vi "TOP-调试与报错.vi"(7 "枚举-错误类型":T1, 8 "错误 i":errorcluster, 11 "输入":variant) -> (0 "错误 o":errorcluster, 3 "输出":variant)   [LabVIEW 2017, in "调试与报错.lvlib"]
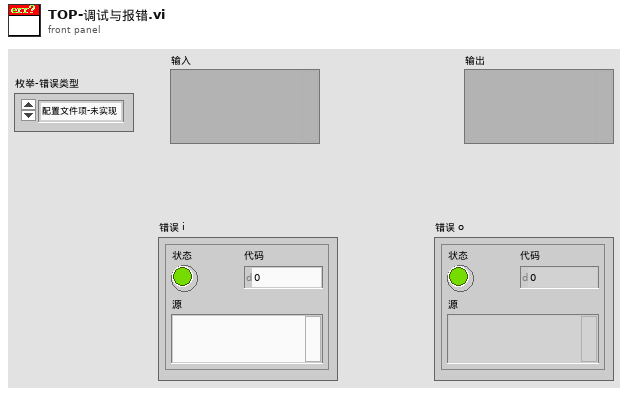
[diagram p1: front panel]
types:
  T1 = typedef "调试与报错.lvlib/枚举-错误类型.ctl" = enum16{"配置文件项-未实现", "路径-未实现"}
  T2 = typedef "调试与报错.lvlib/簇-输入-配置文件项未实现.ctl" = cluster{"段名":string, "键名":string}
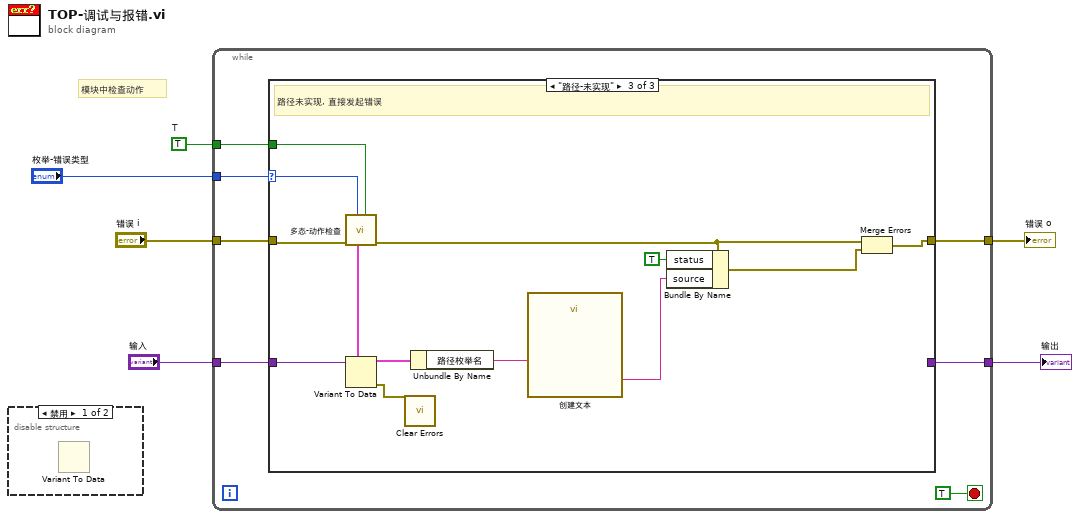
[diagram p0: block diagram]
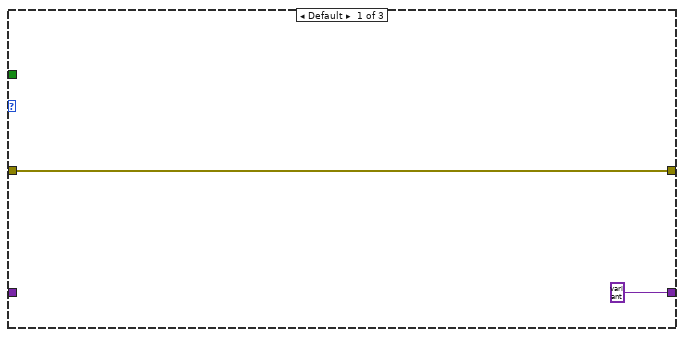
[diagram p3: hidden frame]
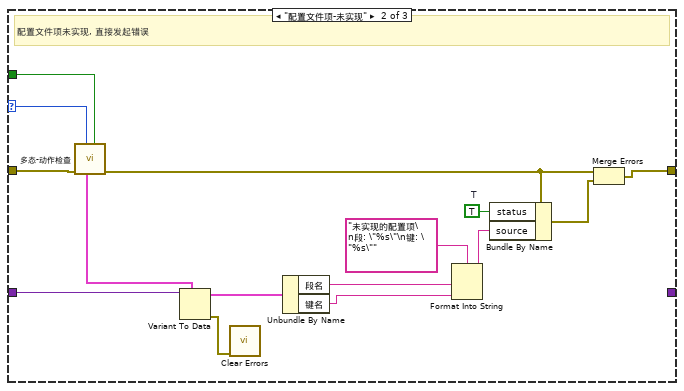
[diagram p4: hidden frame]
diagram:
  w1 = TRUE  # T
  # "模块中检查动作"
  n1 = disable-structure shown="禁用" {
    frame Disabled {
      n2 = Variant To Data() -> ()  [unwired: 3 in, 2 out]
    }
    frame Enabled {
    }
  }
  n3 = while {
    tunnel: "错误 i" -> [w12]
    tunnel: [w11] -> w5
    tunnel: [w10] -> w4
    tunnel: "输入" -> [w9]
    tunnel: "枚举-错误类型" -> [w8]
    tunnel: w1 -> [w7]
    stop <- TRUE stop-if-true
    n4 = case shown="\"路径-未实现\"" w8 {
      selector: w8 -> [_ w17 w34]
      tunnel: w12 -> [w15 w24 w43]
      tunnel: [w15 w25 w37] -> w11
      tunnel: [variant ("输入") _ _] -> w10
      tunnel: w9 -> [_ w30 w42]
      tunnel: w7 -> [_ w16 w33]
      frame Default {
      }
      frame "配置文件项-未实现" {
        w27 = TRUE  # T
        # "配置文件项未实现, 直接发起错误"
        n5 = call-poly "多态-动作检查.vi"("检查动作?"=w16, "枚举-错误类型"=w17, "错误输入"=w24) -> ("错误输出"=w18:errorcluster, "输入"=w23:T2)  [unwired: 6 in, 1 out]
        n6 = Variant To Data(type=w23, Variant=w30) -> (data=w22:T2, error out=w29:errorcluster)  [unwired: 1 in]
        n7 = call <vilib>:"Clear Errors.vi"("error in (no error)"=w29) -> ()  [unwired: 5 in, 2 out]
        n8 = Unbundle By Name(w22) -> ("段名"=w21:string, "键名"=w20:string)
        n9 = Format Into String(format string="未实现的配置项\n段: \"%s\"\n键: \"%s\"" ("格式字符串"), w21, w20) -> (resulting string=w26:string)  [unwired: 2 in, 1 out]
        n10 = Bundle By Name(cluster=w18, "status"=w27, "source"=w26) -> (w19:errorcluster)
        n11 = Merge Errors(w18, w19) -> (w25:errorcluster)
      }
      frame "路径-未实现" {
        # "路径未实现, 直接发起错误"
        n12 = call-poly "多态-动作检查.vi"("检查动作?"=w33, "枚举-错误类型"=w34, "错误输入"=w43) -> ("错误输出"=w36:errorcluster, "输入"=w32:cluster{"路径枚举名":string})  [unwired: 6 in, 1 out]
        n13 = Variant To Data(type=w32, Variant=w42) -> (data=w41:cluster{"路径枚举名":string}, error out=w38:errorcluster)  [unwired: 1 in]
        n14 = call <vilib>:"Clear Errors.vi"("error in (no error)"=w38) -> ()  [unwired: 5 in, 2 out]
        n15 = Unbundle By Name(w41) -> ("路径枚举名"=w31:string)
        n16 = call "创建文本"("路径枚举名"=w31) -> ("Result"=w39:string)  [unwired: 13 in, 1 out]
        n17 = Bundle By Name(cluster=w36, "status"=TRUE, "source"=w39) -> (w35:errorcluster)
        n18 = Merge Errors(w36, w35) -> (w37:errorcluster)
      }
    }
  }
  "输出" <- w4
  "错误 o" <- w5
